vi "Load Signal List.vi"(8 "error in (no error)":errorcluster, 11 "Configuration in":refnum<class "Configuration.lvclass">) -> (0 "error out":errorcluster, 3 "Configuration out":refnum<class "Configuration.lvclass">)   [LabVIEW 2023, in "Configuration.lvlib" / "Configuration.lvclass"]
doc: "Read Signals.csv raw data into memory for reference."
uses:
  Library/Configuration.lvclass
  Library/Configuration.lvclass/Configuration.ctl
  <vilib>/Utility/file.llb/Read Delimited Spreadsheet (string).vi
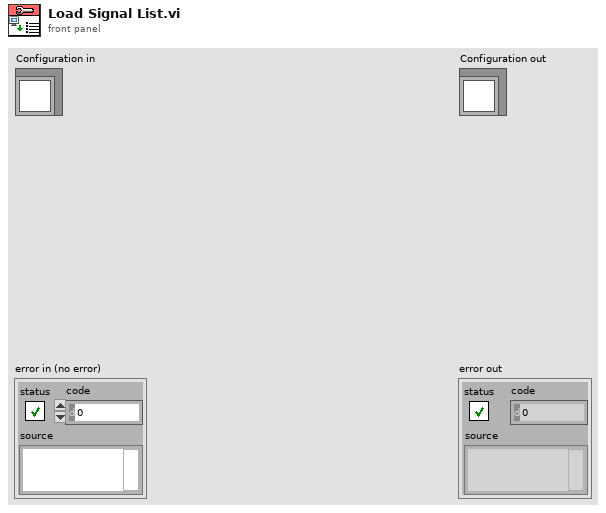
[diagram p1: front panel]
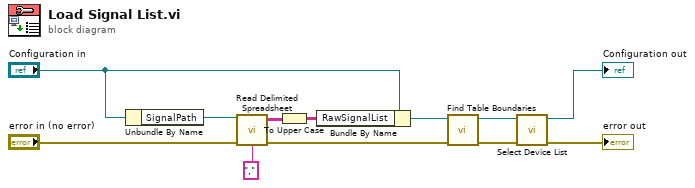
[diagram p0: block diagram]
diagram:
  n1 = Unbundle By Name("Configuration in") -> ("SignalPath"=w12:path)
  n2 = call-poly <vilib>:"Read Delimited Spreadsheet.vi"("file path (dialog if empty)"=w12, "error in (no error)"="error in (no error)", "delimiter (\\t)"="," ("delimiter (\\t)")) -> ("all rows"=w9:string[][], "error out"=w3:errorcluster)  [unwired: 7 in, 4 out]
  n3 = To Upper Case(1:w9) -> (0:w7:string[][])
  n4 = Bundle By Name(cluster="Configuration in", "RawSignalList"=w7) -> (w4:refnum<class "Configuration.lvclass">)
  n5 = call "Find Table Boundaries.vi"("error in (no error)"=w3, "Configuration in"=w4) -> ("error out"=w6:errorcluster, "Configuration out"=w5:refnum<class "Configuration.lvclass">)  [unwired: 8 in]
  n6 = call "Select Device List.vi"("error in (no error)"=w6, "Configuration in"=w5) -> ("error out"=→"error out":errorcluster, "Configuration out"=→"Configuration out":refnum<class "Configuration.lvclass">)  [unwired: 8 in]
